vi "Write DAQ Parameters.vi"(8 "error in (no error)":errorcluster, 10 "DAQ Parameters":T1, 11 "ATS9350 in":refnum<class "ATS9350.lvclass">) -> (0 "error out":errorcluster, 3 "ATS9350 out":refnum<class "ATS9350.lvclass">)   [LabVIEW 2015, in "ATS9350.lvclass"]
uses:
  ATS9350.lvclass
  DAQ Parameters.ctl
  Trigger Source.ctl
  Trigger Slope.ctl
  Type Defs/OCT DAQ Channel Data Type.ctl
  Clock Control.ctl
  ATS-VI/ATS_ctl/ATS_Async_Ctrl.ctl
  ATS-VI/ATS_ctl/ATS_Async_Mode.ctl
  ATS-VI/ATS_ctl/ATS_ReadSamples.ctl
  ATS-VI/ATS_ctl/ATS_Async_Setting.ctl
  ATS-VI/ATS_ctl/ClockRate.ctl
  ATS-VI/ATS_ctl/InputCtrl.ctl
  ATS-VI/ATS_ctl/Coupling.ctl
  ATS-VI/ATS_ctl/Range.ctl
  ATS-VI/ATS_ctl/Impedance.ctl
  ATS-VI/ATS_ctl/Bandwidth.ctl
  ATS-VI/ATS_ctl/ATS_Global.ctl
  ATS-VI/ATS_ctl/Record.ctl
  ATS-VI/ATS_ctl/Clock.ctl
  ATS-VI/ATS_ctl/ClockSource.ctl
  ATS-VI/ATS_ctl/ClockEdge.ctl
  ATS-VI/ATS_ctl/Trigger.ctl
  ATS-VI/ATS_ctl/TriggerOperation.ctl
  ATS-VI/ATS_ctl/TriggerEngine.ctl
  ATS-VI/ATS_ctl/ExtTrigger.ctl
  ATS-VI/ATS_ctl/ExtTrigRange.ctl
  ATS9350.lvclass/ATS9350.ctl
  ATS-VI/ATS_ctl/ATS_DMA_Channel.ctl
  DAQ Class.lvclass
panel:
  out "Return Code":u32
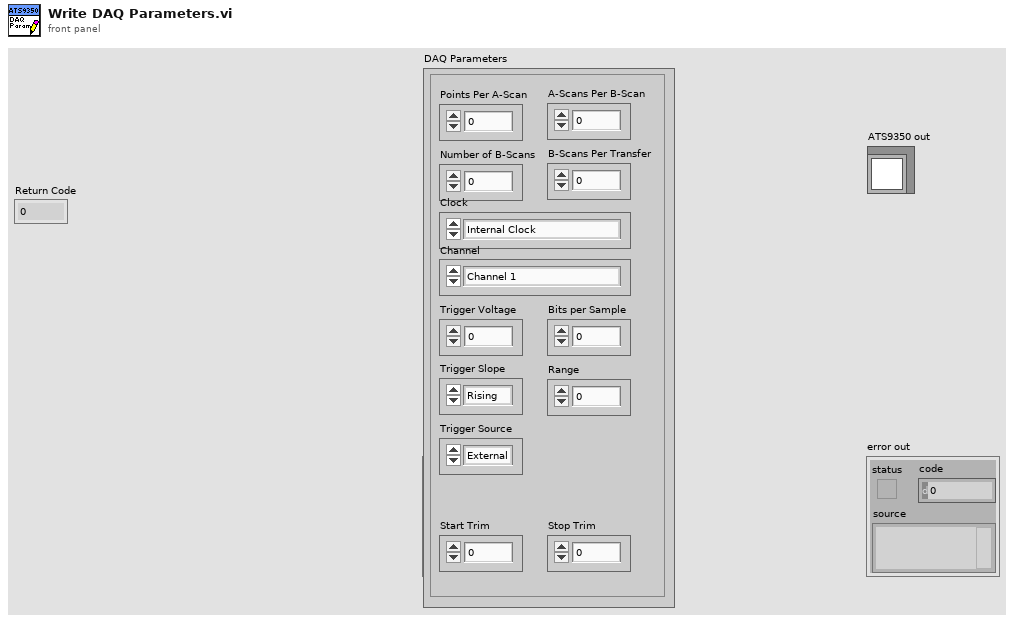
[diagram p1: front panel]
types:
  T1 = typedef "DAQ Class.lvclass/DAQ Parameters.ctl" = cluster{"Points Per A-Scan":u32, "A-Scans Per B-Scan":u32, "Number of B-Scans":u32, "B-Scans Per Transfer":u32, "Trigger Voltage":sgl, "Trigger Source":T2, "Trigger Slope":T3, "Channel":T4, "Clock":T5, "Bits per Sample":dbl, "Range":dbl, "Start Trim":u32, "Stop Trim":u32}
  T2 = typedef "DAQ Class.lvclass/Trigger Source.ctl" = enum16{"External", "Channel A", "Channel B"}
  T3 = typedef "DAQ Class.lvclass/Trigger Slope.ctl" = enum16{"Rising", "Falling"}
  T4 = typedef "OCT DAQ Channel Data Type.ctl" = enum16{"Channel 1", "Channel 2", "Channel 1 and 2"}
  T5 = typedef "DAQ Class.lvclass/Clock Control.ctl" = enum16{"Internal Clock", "External Clock"}
  T6 = typedef "ATS_Global.ctl" = cluster{"Record":T7, "Clock":T8, "Input A":T12, "Input B":T12, "Trigger":T17}
  T7 = typedef "Record.ctl" = cluster{"Count":u32, "Presize":u32, "Length":u32}
  T8 = typedef "Clock.ctl" = cluster{"ClckSource":T9, "ClckRate":T10, "ClckEdge":T11, "Decimation":u32}
  T9 = typedef "ClockSource.ctl" = enum16{"Internal", "External", "Medium Ext.", "Slow Ext.", "Ext. AC", "Ext. DC", "Ext. (PLL)"}
  T10 = typedef "ClockRate.ctl" = u32
  T11 = typedef "ClockEdge.ctl" = u16
  T12 = typedef "InputCtrl.ctl" = cluster{"Coupling":T13, "Range":T14, "Impedance":T15, "Bandwidth":T16}
  T13 = typedef "Coupling.ctl" = enum16{"AC", "DC"}
  T14 = typedef "Range.ctl" = u32
  T15 = typedef "Impedance.ctl" = enum16{"1M ohms", "50 ohms"}
  T16 = typedef "Bandwidth.ctl" = enum16{"Full Bandwidth", "Reduce Bandwidth"}
  T17 = typedef "Trigger.ctl" = cluster{"TrigOperation":T18, "Timeout (s)":dbl, "Trig. Delay":u32, "Engine X":T19, "Engine Y":T19, "ExtTrigControl":T20}
  T18 = typedef "TriggerOperation.ctl" = enum16{"Only X", "Only Y", "X or Y", "X and Y", "X xor Y", "X and not Y", "not X and Y"}
  T19 = typedef "TriggerEngine.ctl" = cluster{"Source":enum32{"Chan_A", "Chan_B", "External", "Disable"}, "Slope":enum32{"Positive", "Negative"}, "Level":u32}
  T20 = typedef "ExtTrigger.ctl" = cluster{"Coupling":T13, "Range":T21}
  T21 = typedef "ExtTrigRange.ctl" = enum16{"1 V", "5 V", "TTL"}
  T22 = typedef "ATS_Async_Setting.ctl" = cluster{"UseHeader":u32, "Rec/Buffer":u32, "Total_Rec":u32, "DataBuffer":bool, "GetProcessedData":bool}
  T23 = typedef "ATS_ReadSamples.ctl" = cluster{"Offset":i32, "Length":u32}
  T24 = typedef "ATS_Async_Mode.ctl" = enum16{"Continuous", "Triggered", "No-Pre-Trigger", "Traditional"}
  T25 = typedef "ATS_Async_Ctrl.ctl" = enum16{"SetupDMA", "StartCapture", "Get", "Get_Stream", "Abort", "Stop"}
  T26 = enum32{"Chan_A", "Chan_B", "External", "Disable"}
  T27 = typedef "ATS_DMA_Channel.ctl" = enum16{"Channel_A", "Channel_B", "A & B"}
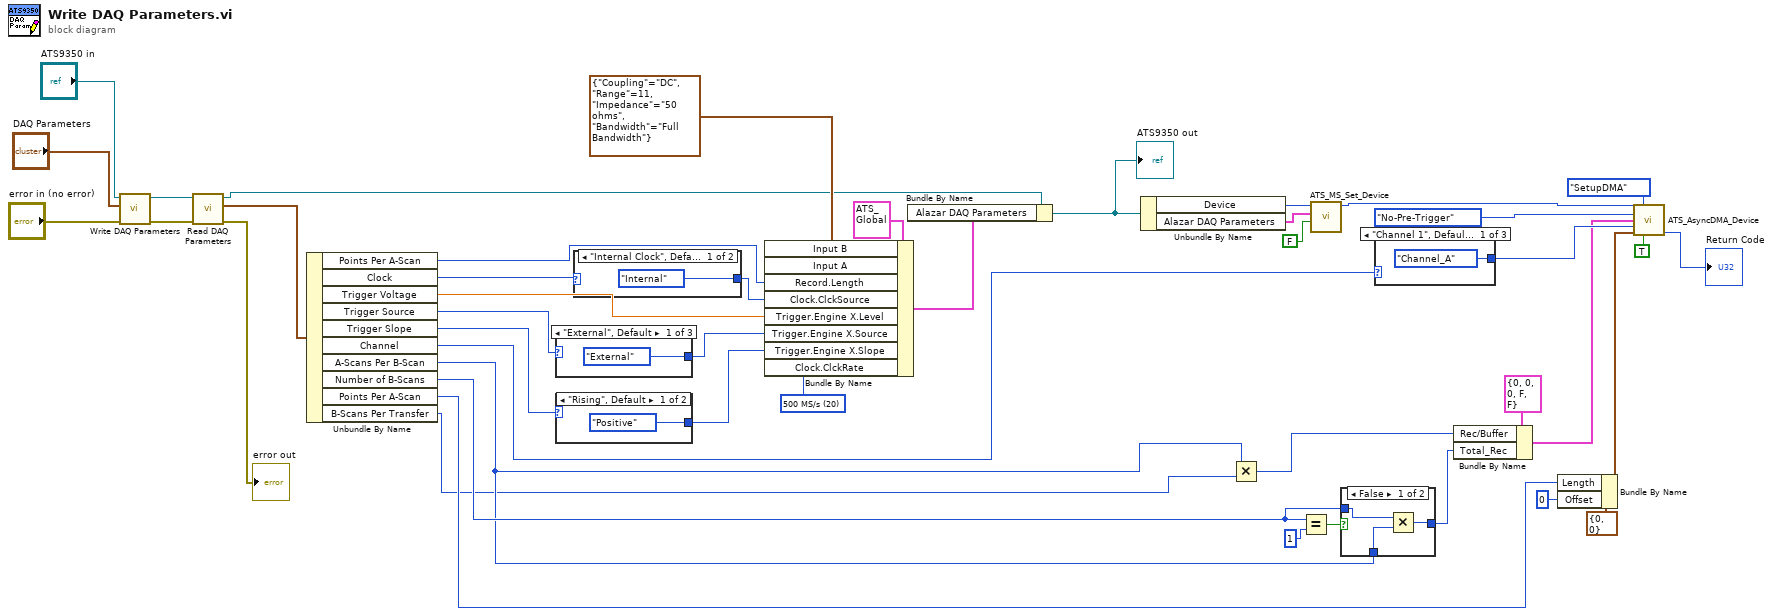
[diagram p0: block diagram]
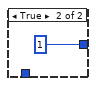
[diagram p2: hidden frame]
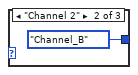
[diagram p3: hidden frame]
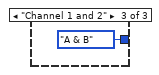
[diagram p4: hidden frame]
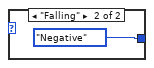
[diagram p5: hidden frame]
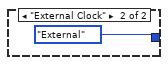
[diagram p6: hidden frame]
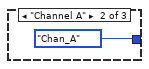
[diagram p7: hidden frame]
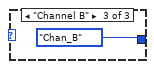
[diagram p8: hidden frame]
diagram:
  w12 = T12 {"Coupling"=enum."DC", "Range"=11, "Impedance"=enum."50 ohms", "Bandwidth"=enum."Full Bandwidth"} ("Input A")
  w15 = T10 20 items=["1 kS/s", "2 kS/s", "5 kS/s", "10 kS/s", "20 kS/s", "50 kS/s", "100 kS/s", "200 kS/s", "500 kS/s", "1 MS/s", "2 MS/s", "5 MS/s", "10 MS/s", "20 MS/s", "25 MS/s", "50 MS/s", "100 MS/s", "125 MS/s", "200 MS/s", "250 MS/s", "500 MS/s", "1 GS/s"] ("Clock.ClckRate")
  n1 = call-parent "Write DAQ Parameters.vi"("error in (no error)"="error in (no error)", "DAQ Parameters"="DAQ Parameters", "DAQ Class in"="ATS9350 in") -> ("error out"=w8:errorcluster, "DAQ Class out"=w9:refnum<class "ATS9350.lvclass">)  [unwired: 7 in]
  n2 = call-dynamic "Read DAQ Parameters.vi"("error in (no error)"=w8, "ATS9350 in"=w9) -> ("error out"=→"error out":errorcluster, "DAQ Parameters"=w16:T1, "ATS9350 out"=w11:refnum<class "ATS9350.lvclass">)  [unwired: 7 in]
  n3 = Unbundle By Name(w16) -> ("Points Per A-Scan"=w39:u32, "Clock"=w38:T5, "Trigger Voltage"=w36:sgl, "Trigger Source"=w41:T2, "Trigger Slope"=w35:T3, "Channel"=w4:T4, "A-Scans Per B-Scan"=w3:u32, "Number of B-Scans"=w6:u32, "Points Per A-Scan"=w5:u32, "B-Scans Per Transfer"=w1:u32)
  n4 = case shown="\"External\", Default" w41 {
    tunnel: [T26."External" ("Trigger.Engine X.Source") T26."Chan_A" ("Trigger.Engine X.Source") T26."Chan_B" ("Trigger.Engine X.Source")] -> w40
    frame "External", Default {
    }
    frame "Channel A" {
    }
    frame "Channel B" {
    }
  }
  n5 = case shown="\"Rising\", Default" w35 {
    tunnel: [enum32{"Positive", "Negative"}."Positive" ("Trigger.Engine X.Slope") enum32{"Positive", "Negative"}."Negative" ("Trigger.Engine X.Slope")] -> w34
    frame "Rising", Default {
    }
    frame "Falling" {
    }
  }
  n6 = case shown="\"Internal Clock\", Default" w38 {
    tunnel: [ClockSource."Internal" ("Clock.ClckSource") ClockSource."External" ("Clock.ClckSource")] -> w37
    frame "Internal Clock", Default {
    }
    frame "External Clock" {
    }
  }
  n7 = Bundle By Name(cluster=T6 {"Record"={"Count"=0, "Presize"=0, "Length"=0}, "Clock"={"ClckSource"=enum."Internal", "ClckRate"=0, "ClckEdge"=0, "Decimation"=0}, "Input A"={"Coupling"=enum."DC", "Range"=12, "Impedance"=enum."1M ohms", "Bandwidth"=enum."Full Bandwidth"}, "Input B"={"Coupling"=enum."DC", "Range"=12, "Impedance"=enum."1M ohms", "Bandwidth"=enum."Full Bandwidth"}, "Trigger"={"TrigOperation"=enum."Only X", "Timeout (s)"=-1.0, "Trig. Delay"=0, "Engine X"={"Source"=enum."Chan_A", "Slope"=enum."Positive", "Level"=0}, "Engine Y"={"Source"=enum."Chan_A", "Slope"=enum."Positive", "Level"=0}, "ExtTrigControl"={"Coupling"=enum."DC", "Range"=enum."1 V"}}} ("Value"), "Input B"=w12, "Input A"=w12, "Record.Length"=w39, "Clock.ClckSource"=w37, "Trigger.Engine X.Level"=w36, "Trigger.Engine X.Source"=w40, "Trigger.Engine X.Slope"=w34, "Clock.ClckRate"=w15) -> (w27:T6)
  n8 = Bundle By Name(cluster=w11, "Alazar DAQ Parameters"=w27) -> (w7:refnum<class "ATS9350.lvclass">)
  "ATS9350 out" <- w7
  n9 = Unbundle By Name(w7) -> ("Device"=w25:i32, "Alazar DAQ Parameters"=w24:T6)
  n10 = Multiply(x=w3, y=w1) -> (x*y=w2:u32)
  n11 = Equal?(x=w6, y=u32 1) -> (x = y?=w18:bool)
  n12 = call "ATS_MS_Set_Device.vi"("Set_Manually (F)"=FALSE, "Setup_In"=w24, "DeviceIn"=w25) -> ("DeviceOut"=w14:i32)  [unwired: 3 in, 5 out]
  n13 = case shown="False" w18 {
    tunnel: [w54 u32 1 ("y")] -> w17
    tunnel: w3 -> [w53 _]
    tunnel: w6 -> [w52 _]
    frame False {
      n14 = Multiply(x=w52, y=w53) -> (x*y=w54:u32)
    }
    frame True {
    }
  }
  n15 = case shown="\"Channel 1\", Default" w4 {
    tunnel: [ATS_DMA_Channel."Channel_A" ("Channel") ATS_DMA_Channel."Channel_B" ("Channel") ATS_DMA_Channel."A & B" ("Channel")] -> w33
    frame "Channel 1", Default {
    }
    frame "Channel 2" {
    }
    frame "Channel 1 and 2" {
    }
  }
  n16 = Bundle By Name(cluster=T22 {"UseHeader"=0, "Rec/Buffer"=0, "Total_Rec"=0, "DataBuffer"=FALSE, "GetProcessedData"=FALSE} ("Async_Setting"), "Rec/Buffer"=w2, "Total_Rec"=w17) -> (w21:T22)
  n17 = Bundle By Name(cluster=T23 {"Offset"=0, "Length"=0} ("ReadSamples"), "Length"=w5, "Offset"=0) -> (w31:T23)
  n18 = call "ATS_AsyncDMA_Device.vi"("DeviceIn"=w14, "ATS_Async_Ctrl"=ATS_Async_Ctrl."SetupDMA" ("ATS_DMA_Ctrl"), "Async_Mode"=ATS_Async_Mode."No-Pre-Trigger", "Async_Setting"=w21, "Channel"=w33, "ReadSamples"=w31, "Start Now / Wait"=TRUE) -> ("Return Code"=→"Return Code":u32)  [unwired: 4 in, 4 out]
